vi "Load Configuration File.vi"(8 "error in":errorcluster, 10 "Filename":string, 11 "Bobcat 640 in":refnum<class "Bobcat 640.lvclass">) -> (0 "error out":errorcluster, 2 "Supported?":bool, 3 "Bobcat 640 out":refnum<class "Bobcat 640.lvclass">)   [LabVIEW 2018, in "Bobcat 640.lvlib" / "Bobcat 640.lvclass"]
uses:
  Bobcat 640.lvclass
  Bobcat 640.lvclass/Bobcat 640.ctl
  c0553d17-b2ab-46ef-9008-45d403a28afc.vi
  <resource>/objmgr/imaqdx.rc
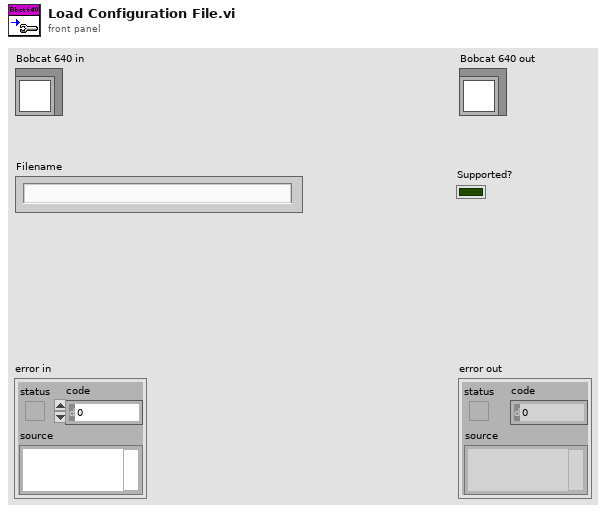
[diagram p1: front panel]
types:
  T1 = typedef "IMAQdx.ctl" = refnum<k21>
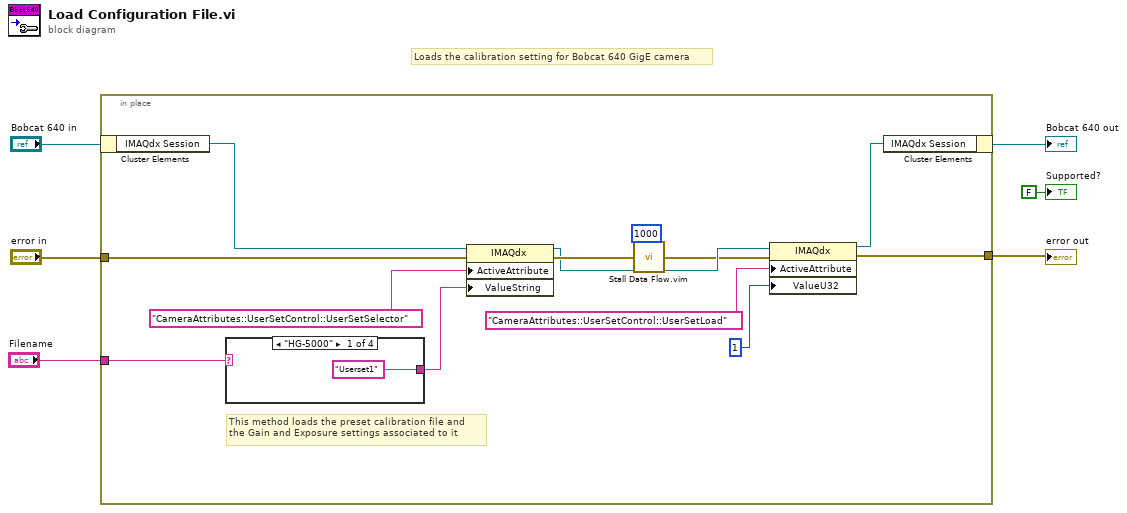
[diagram p0: block diagram]
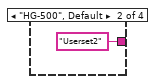
[diagram p2: hidden frame]
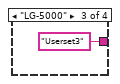
[diagram p3: hidden frame]
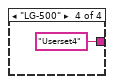
[diagram p4: hidden frame]
diagram:
  # "Loads the calibration setting for Bobcat 640 GigE camera"
  n1 = in-place {
    in-place-border: "Filename" -> [w11]
    in-place-border: "error in" -> [w9]
    in-place-border: [w7] -> w1
    # "This method loads the preset calibration file and \nthe Gain and Exposure settings associated to it"
    n2 = in-place-cluster #1("Bobcat 640 in") -> ("IMAQdx Session"=w15:T1)
    n3 = case shown="\"HG-5000\"" w11 {
      tunnel: ["Userset1" "Userset2" "Userset3" "Userset4"] -> w16
      frame "HG-5000" {
      }
      frame "HG-500", Default {
      }
      frame "LG-5000" {
      }
      frame "LG-500" {
      }
    }
    n4 = property class="IMAQdx"(reference=w15, error in=w9, "ActiveAttribute"="CameraAttributes::UserSetControl::UserSetSelector", "ValueString"=w16) -> (reference out=w14:T1, error out=w18:errorcluster)
    n5 = call "Stall Data Flow.vim"("value in"=w18, "milliseconds to wait"=u32 1000) -> ("value out"=w8:errorcluster)  [unwired: 1 out]
    n6 = property class="IMAQdx"(reference=w14, error in=w8, "ActiveAttribute"="CameraAttributes::UserSetControl::UserSetLoad", "ValueU32"=u32 1) -> (reference out=w10:T1, error out=w7:errorcluster)
    n7 = in-place-cluster #1("IMAQdx Session"=w10) -> (→"Bobcat 640 out":refnum<class "Bobcat 640.lvclass">)
  }
  "error out" <- w1
  "Supported?" <- FALSE ("Supported?")
